vi "Create Directories.vi"(8 "error in (no error)":errorcluster, 11 "Kasli Wrapper 2.0 in":refnum<class "Kasli Wrapper 2.0.lvclass">) -> (0 "error out":errorcluster, 3 "Kasli Wrapper 2.0 out":refnum<class "Kasli Wrapper 2.0.lvclass">)   [LabVIEW 2020, in "Kasli Wrapper 2.0.lvlib" / "Kasli Wrapper 2.0.lvclass"]
uses:
  Kasli Wrapper 2.0.lvclass
  Kasli Wrapper 2.0.lvclass/Kasli Wrapper 2.0.ctl
  Ancestor/Ancestor/Ancestor.lvclass/Ancestor.ctl
  Support VIs/Generate Error.vi
  FGV/Error Memory/Get Error Description.vi
  Support VIs/Get PC name.vi
  Ancestor/Ancestor/Read ID.vi
  Support VIs/Get Class Name.vi
  <vilib>/Utility/error.llb/Clear Errors.vi
  FGV/Error Memory/Error Memory Core.vi
  <vilib>/AdvancedString/Delimited String to 1D String Array.vi
  Support VIs/Circus Root Path.vi
  FGV/Error Memory/Error Crt Lvl checker.vi
  FGV/Error Memory/Error Memory Core.vi/40c8088d-b597-4017-91af-faa98e00292e.vi
  FGV/Error Memory/Error Memory Core.vi/d4a3ab98-063c-4e44-b43d-fbdcfe6c2be2.vi
  Support VIs/Global Memory.vi
  <vilib>/Utility/LVClass/Get LV Class Name.vi
  Support VIs/Is in Packed Library.vi
  Support VIs/TALOS Root path.vi
  Support VIs/Read CSV worksheet.vi
  Support VIs/Global Constants.vi
  <vilib>/Utility/error.llb/General Error Handler.vi
  Support VIs/Error Log.vi
  Ancestor/Ancestor/Ancestor.lvclass
  <vilib>/Comparison/Equal/Equal Functor/Equal Functor.lvclass
  TALOS.lvlib
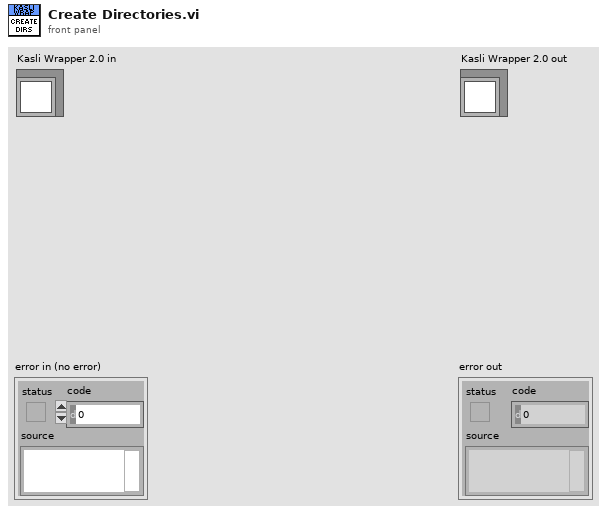
[diagram p1: front panel]
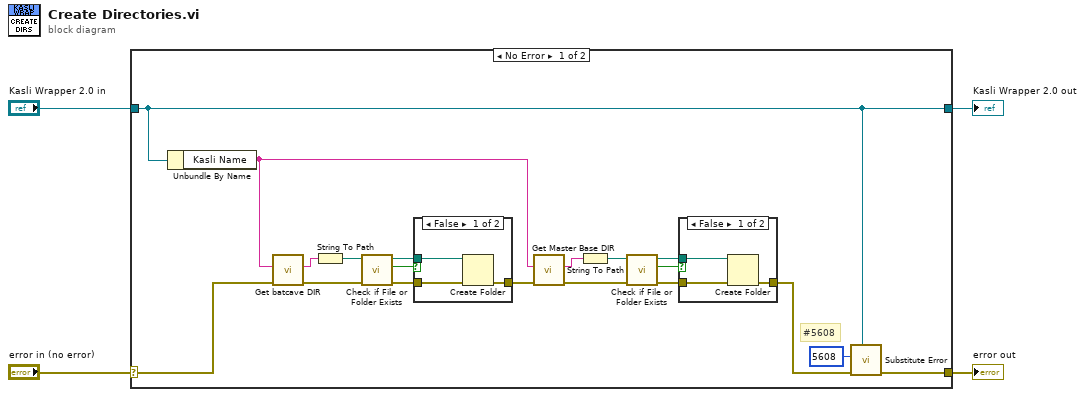
[diagram p0: block diagram]
diagram:
  n1 = case shown="No Error" "error in (no error)" {
    selector: "error in (no error)" -> [w23 w33]
    tunnel: [w18 w33] -> w3
    tunnel: [w17 w32] -> w1
    tunnel: "Kasli Wrapper 2.0 in" -> [w17 w32]
    frame No Error {
      # "#5608"
      n2 = Unbundle By Name(w17) -> ("Kasli Name"=w7:string)
      n3 = call "Get batcave DIR.vi"("error in (no error)"=w23, "relative path"=w7) -> ("error out"=w22:errorcluster, "Batcave DIR"=w15:string)  [unwired: 4 in]
      n4 = String To Path(string=w15) -> (path=w20:path)
      n5 = call <vilib>:"Check if File or Folder Exists.vi"("error in (no error)"=w22, "path"=w20) -> ("error out"=w19:errorcluster, "file or folder exists?"=w21:bool, "dup path"=w5:path)  [unwired: 7 in]
      n6 = case shown="False" w21 {
        tunnel: w5 -> [w30 _]
        tunnel: w19 -> [w29 w31]
        tunnel: [w28 w31] -> w10
        frame False {
          n7 = Create Folder(path (use dialog)=w30, error in=w29) -> (error out=w28:errorcluster)  [unwired: 1 in, 2 out]
        }
        frame True {
        }
      }
      n8 = call "Get Master Base DIR.vi"("error in (no error)"=w10, "relative path"=w7) -> ("error out"=w9:errorcluster, "Master DIR"=w8:string)  [unwired: 4 in]
      n9 = String To Path(string=w8) -> (path=w13:path)
      n10 = call <vilib>:"Check if File or Folder Exists.vi"("error in (no error)"=w9, "path"=w13) -> ("error out"=w14:errorcluster, "file or folder exists?"=w12:bool, "dup path"=w6:path)  [unwired: 7 in]
      n11 = case shown="False" w12 {
        tunnel: w6 -> [w26 _]
        tunnel: w14 -> [w25 w27]
        tunnel: [w24 w27] -> w11
        frame False {
          n12 = Create Folder(path (use dialog)=w26, error in=w25) -> (error out=w24:errorcluster)  [unwired: 1 in, 2 out]
        }
        frame True {
        }
      }
      n13 = call "Substitute Error.vi"("LabVIEW Object"=w17, "error in (no error)"=w11, "Error Code"=5608) -> ("error out"=w18:errorcluster)  [unwired: 8 in]
    }
    frame Error {
    }
  }
  "error out" <- w3
  "Kasli Wrapper 2.0 out" <- w1
